vi "Get subset of CSV.vi"() -> ()   [LabVIEW 2017]
uses:
  <vilib>/Utility/file.llb/Read Delimited Spreadsheet (DBL).vi
  <vilib>/Utility/file.llb/Write Delimited Spreadsheet (DBL).vi
panel:
  in  "append to file? (new file:F)":bool
  in  "index (row)":i32
  in  "File Out":path
  in  "File In":path
  out "Error Out":errorcluster
  in  "Error In":errorcluster
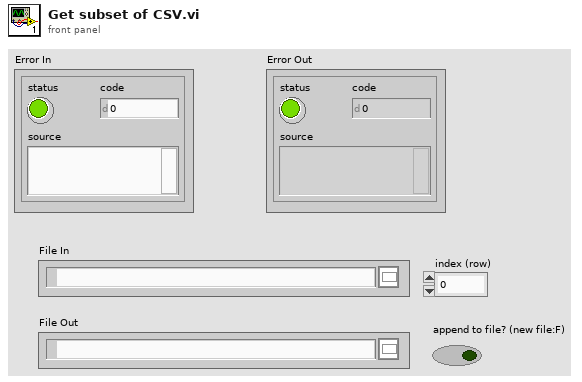
[diagram p1: front panel]
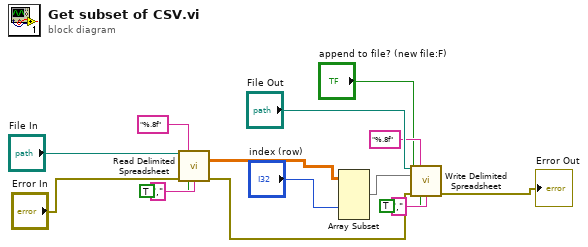
[diagram p0: block diagram]
diagram:
  n1 = call-poly <vilib>:"Read Delimited Spreadsheet.vi"("file path (dialog if empty)"="File In", "format (%.3f)"="%.8f", "error in (no error)"="Error In", "transpose? (F)"=TRUE, "delimiter (\\t)"="," ("delimiter (\\t)")) -> ("all rows"=w11:dbl[][], "error out"=w6:errorcluster)  [unwired: 5 in, 4 out]
  n2 = Array Subset(array=w11, index (col)="index (row)") -> (w10:dbl[][])  [unwired: 3 in]
  n3 = call-poly <vilib>:"Write Delimited Spreadsheet.vi"("file path (dialog if empty)"="File Out", "format (%.3f)"="%.8f", "2D data"=w10, "append to file? (new file:F)"="append to file? (new file:F)", "error in (no error)"=w6, "transpose? (no:F)"=TRUE, "delimiter (\\t)"="," ("delimiter (\\t)")) -> ("error out"=→"Error Out":errorcluster)  [unwired: 7 in, 1 out]
